vi "Facade 1.vi"(0 "Data In":T6, 2 "Display State In":T2={"Panels_Refnums_Array"=[], "Panel_Command"={"Operation"=enum."Add Item", "Data"=variant}}, 3 "Container State":T5) -> (6 "Data Out":T6, 7 "Display State Out":T2={"Panels_Refnums_Array"=[], "Panel_Command"={"Operation"=enum."Add Item", "Data"=variant}}, 8 "Action":T1)   [LabVIEW 2013, in "UI Panels.lvlib" / "Panels_XControl.xctl"]
uses:
  Panels_XControl.xctl
  Data 1.ctl
  <vilib>/_xctls/Container State.ctl
  State 1.ctl
  Controls/References/Panel_Refnums.ctl
  Controls/Panel_Command_Enum.ctl
  <vilib>/_xctls/Action.ctl
  Typedefs/Splitter Properties.ctl
  Typedefs/Menu Event.ctl
  <vilib>/_xctls/XControlSupport.lvlib
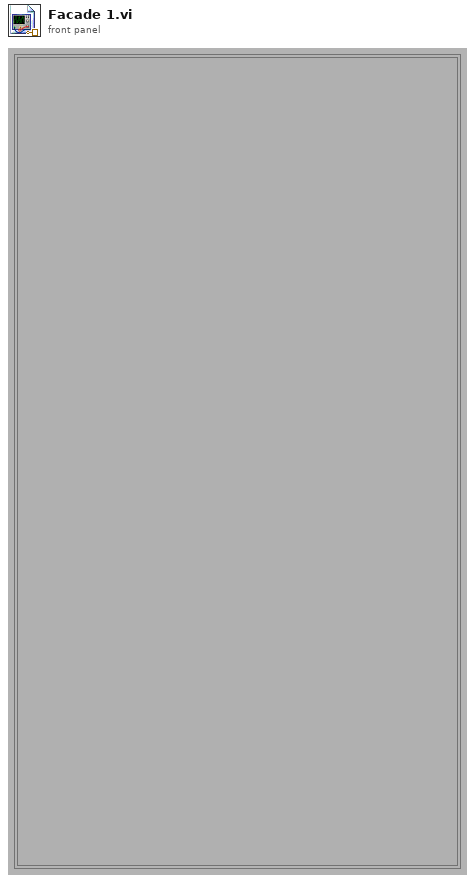
[diagram p1: front panel]
types:
  T1 = typedef "XControlSupport.lvlib/Action.ctl" = cluster{"Data Changed?":bool, "State Changed?":bool, "Action Name":string}
  T2 = typedef "UI Panels.lvlib/Panels_XControl.xctl/State 1.ctl" = cluster{"Panels_Refnums_Array":T3[], "Panel_Command":cluster{"Operation":T4, "Data":variant}}
  T3 = typedef "UI Panels.lvlib/Panels_XControl.xctl/Panel_Refnums.ctl" = cluster{"VI Refnum":refnum<vi>, "Command":refnum<user-event>, "Visible":bool}
  T4 = typedef "UI Panels.lvlib/Panels_XControl.xctl/Panel_Command_Enum.ctl" = enum16{"Idle", "Remove & Stop", "Add Item", "Delete Item", "Delete All", "Insert into Subpanel", "Register Menu Events", "Update Value", "Remove from Subpanel", "Set Title", "Set Menu Items", "Insert SubPanel", "Set Splitter Position", "Set Splitter Properties", "Add Menu Items"}
  T5 = typedef "XControlSupport.lvlib/Container State.ctl" = cluster{"Indicator?":bool, "Run Mode?":bool, " Refnum":refnum<vi>}
  T6 = typedef "UI Panels.lvlib/Panels_XControl.xctl/Data 1.ctl" = refnum<vi>[]
  T7 = typedef "UI Panels.lvlib/Panels_XControl.xctl/Splitter Properties.ctl" = cluster{"index":i32, "Height (Collapsed)":i32, "Height (Expanded)":i32, "Expanded by Default":bool, "Collapsable":bool, "Resizible":bool}
  T8 = typedef "UI Panels.lvlib/Panels_XControl.xctl/Menu Event.ctl" = refnum<user-event>
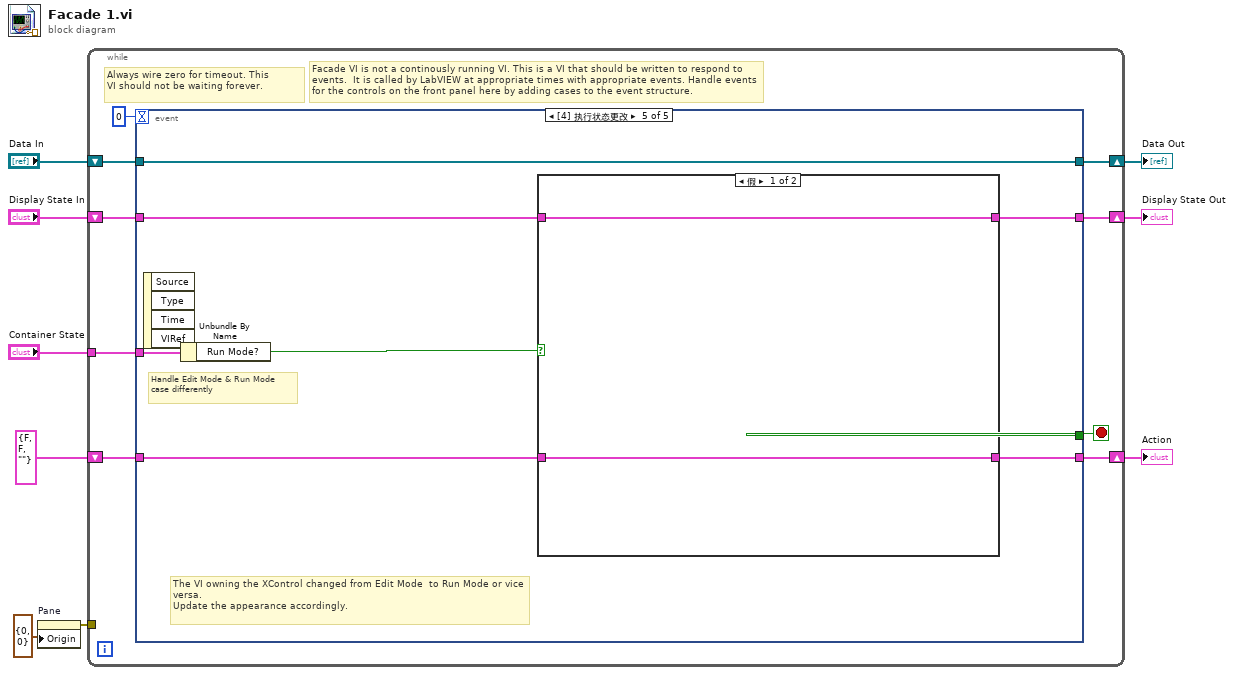
[diagram p0: block diagram]
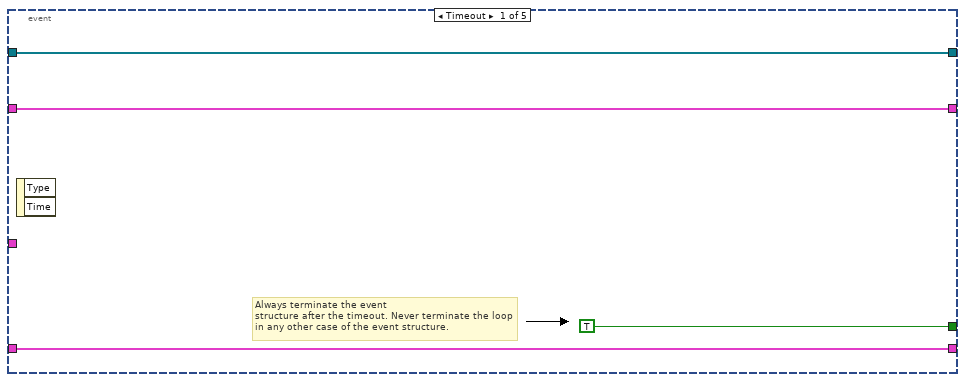
[diagram p2: hidden frame]
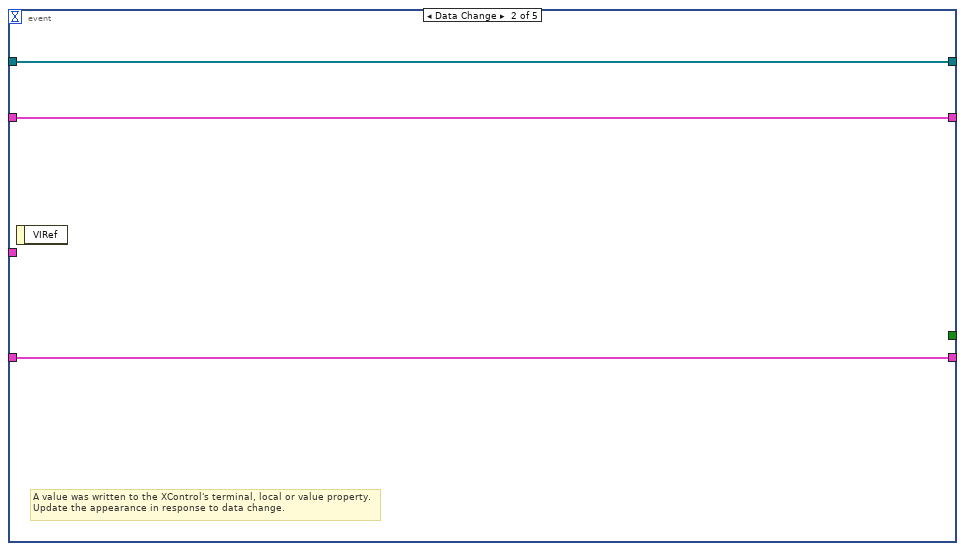
[diagram p3: hidden frame]
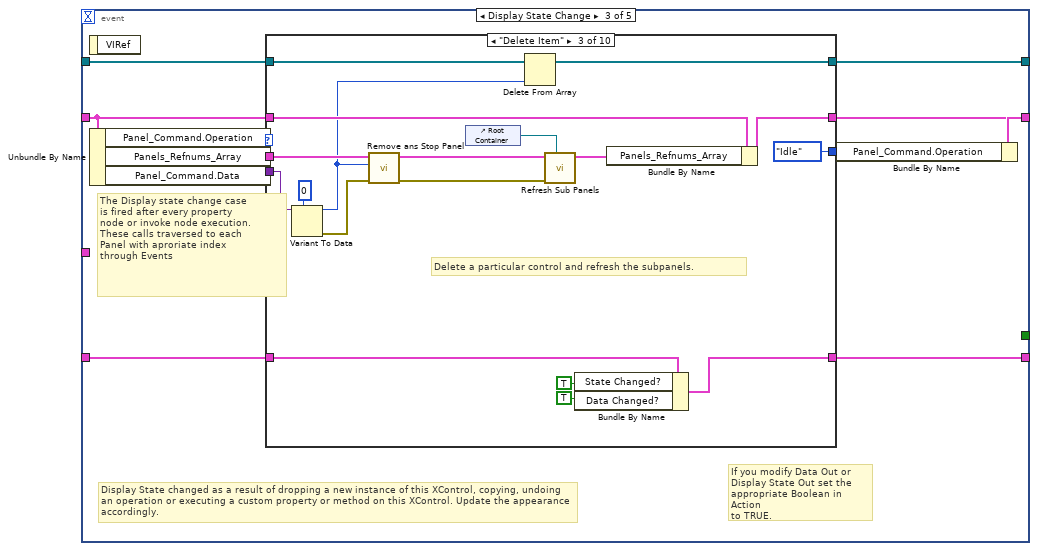
[diagram p4: hidden frame]
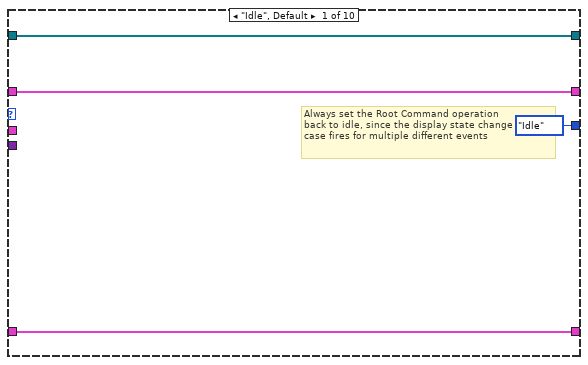
[diagram p5: hidden frame]
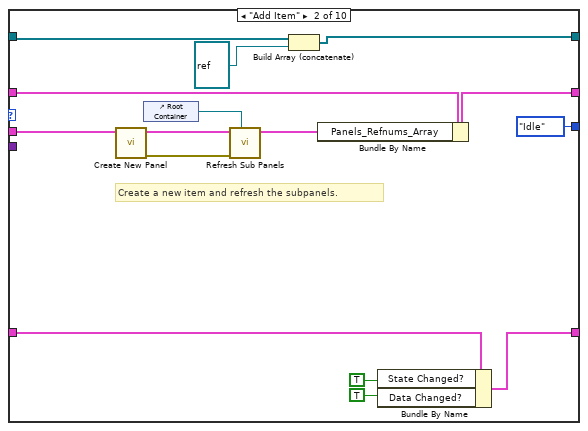
[diagram p6: hidden frame]
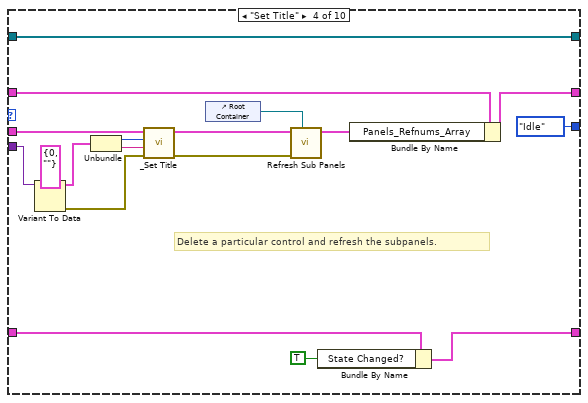
[diagram p7: hidden frame]
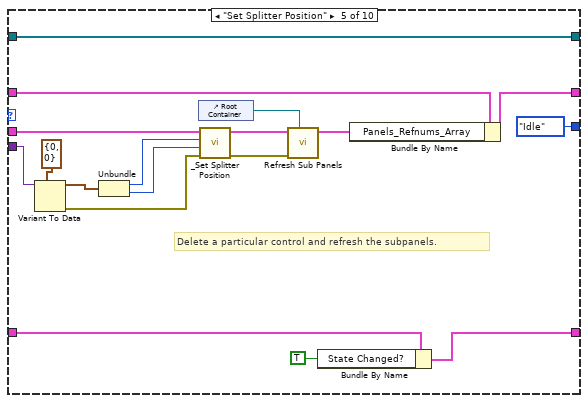
[diagram p8: hidden frame]
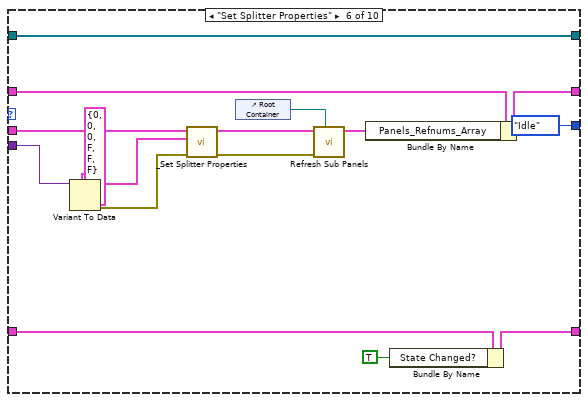
[diagram p9: hidden frame]
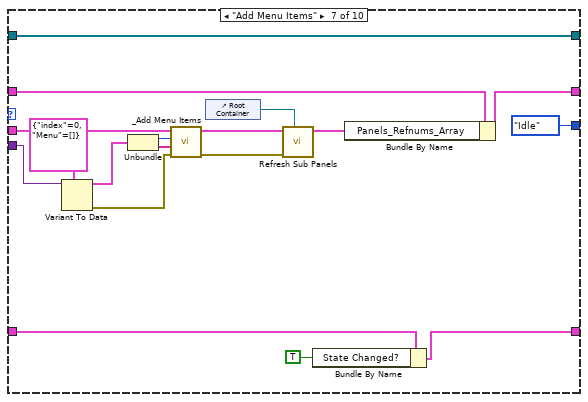
[diagram p10: hidden frame]
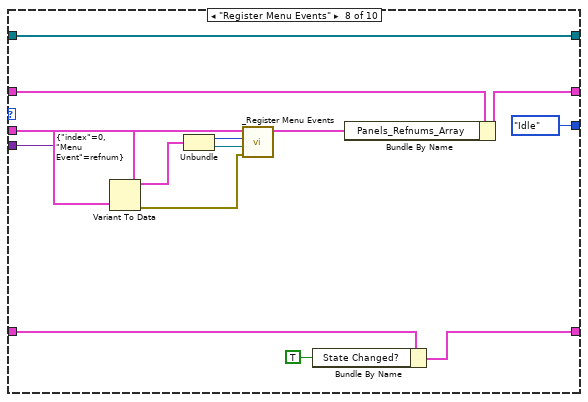
[diagram p11: hidden frame]
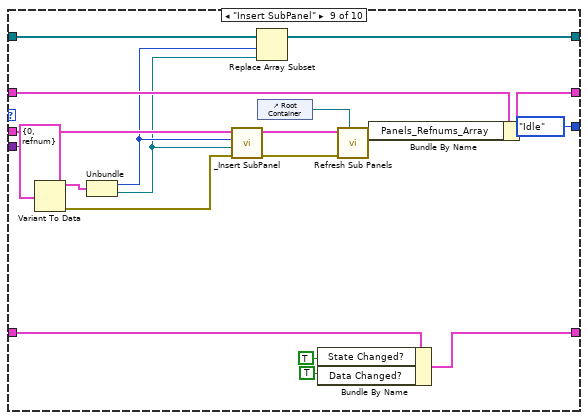
[diagram p12: hidden frame]
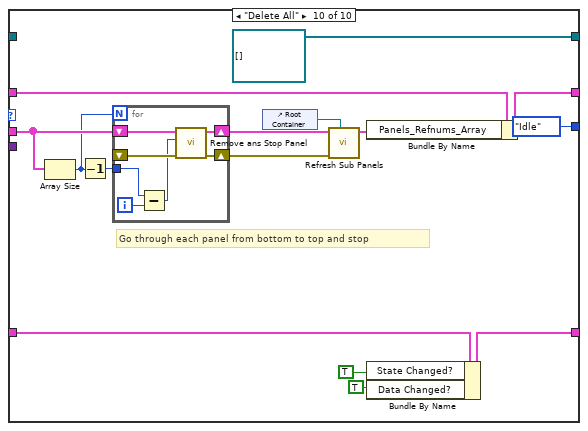
[diagram p13: hidden frame]
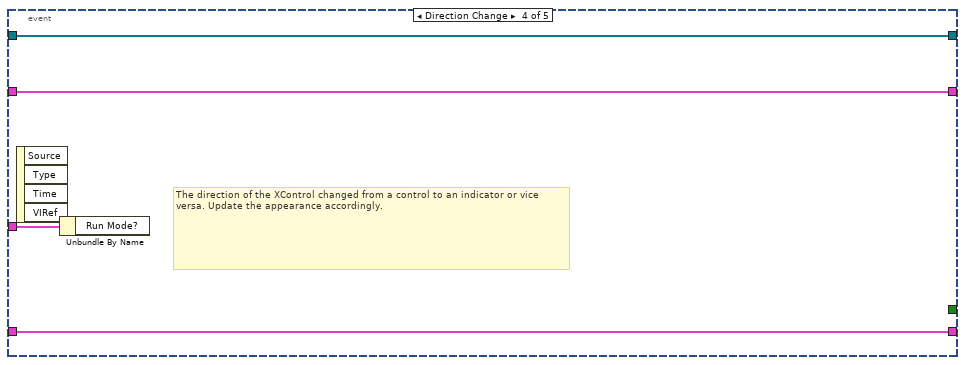
[diagram p14: hidden frame]
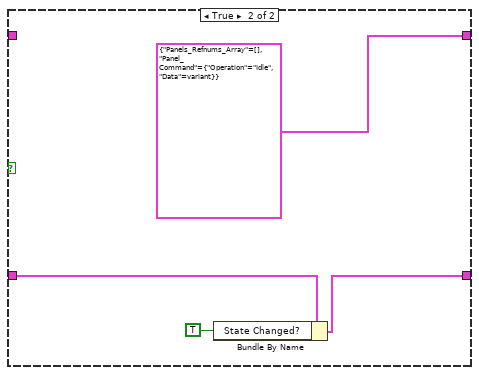
[diagram p15: hidden frame]
diagram:
  n1 = property on="Pane" class="Pane"("Origin"=cluster{"Horizontal":i16, "Vertical":i16} {"Horizontal"=0, "Vertical"=0}) -> (error out=w1:errorcluster)  [unwired: 2 in, 1 out]
  n2 = while {
    shift-right: [w17] -> w3
    shift-left: "Display State In" -> [w18]
    tunnel: "Container State" -> [w14]
    shift-right: [w12] -> w9
    shift-left: "Data In" -> [w13]
    shift-right: [w10] -> w5
    shift-left: T1 {"Data Changed?"=FALSE, "State Changed?"=FALSE, "Action Name"=""} ("Action") -> [w11]
    tunnel: w1 -> [_]
    stop <- w16 stop-if-true
    # "Facade VI is not a continously running VI. This is a VI that should be written to respond to events.  It is called by LabVIEW at appropriate times with appropriate events. Handle events for the controls on the front panel here by adding cases to the event structure."
    # "Always wire zero for timeout. This\nVI should not be waiting forever."
    n3 = event shown="[4] 执行状态更改" {
      selector: _ -> [_ _ _ _ _]
      dyn-events: _ -> [_ _ _ _ _]
      timeout: 0 -> [_ _ _ _ _]
      tunnel: w18 -> [w20 w24 w36 w203 w205]
      tunnel: [w20 w24 w32 w203 w207] -> w17
      tunnel: [TRUE _ _ _ _] -> w16
      tunnel: w14 -> [_ _ _ w204 w211]
      tunnel: w13 -> [w19 w25 w27 w202 w210]
      tunnel: [w19 w25 w26 w202 w210] -> w12
      tunnel: [w21 w23 w33 w201 w208] -> w10
      tunnel: w11 -> [w21 w23 w34 w201 w209]
      event Timeout {
        # "Always terminate the event\nstructure after the timeout. Never terminate the loop in any other case of the event structure."
        n4 = event-data() -> ()  [unwired: 3 out]
      }
      event Data Change {
        # "A value was written to the XControl's terminal, local or value property.\nUpdate the appearance in response to data change."
        n5 = event-data() -> ()  [unwired: 2 out]
      }
      event Display State Change {
        # "If you modify Data Out or\nDisplay State Out set the\nappropriate Boolean in Action\nto TRUE."
        # "The Display state change case\nis fired after every property\nnode or invoke node execution.\nThese calls traversed to each\nPanel with aproriate index\nthrough Events"
        # "Display State changed as a result of dropping a new instance of this XControl, copying, undoing an operation or executing a custom property or method on this XControl. Update the appearance accordingly."
        n6 = event-data() -> ()  [unwired: 2 out]
        n7 = Unbundle By Name(w36) -> ("Panel_Command.Operation"=w35:T4, "Panels_Refnums_Array"=w30:T3[], "Panel_Command.Data"=w29:variant)
        n8 = case shown="\"Delete Item\"" w35 {
          tunnel: w36 -> [w40 w55 w72 w91 w109 w120 w138 w156 w178 w188]
          tunnel: w34 -> [w39 w52 w70 w89 w107 w112 w134 w152 w176 w193]
          tunnel: [w40 w54 w71 w90 w108 w119 w137 w155 w177 w186] -> w31
          tunnel: [w39 w51 w68 w87 w105 w117 w135 w153 w174 w191] -> w33
          tunnel: w30 -> [_ w49 w65 w84 w102 w116 w133 w151 w171 w181]
          tunnel: w29 -> [_ _ w67 w86 w104 w115 w132 w150 w173 _]
          tunnel: [Panel_Command_Enum."Idle" ("Operation") Panel_Command_Enum."Idle" ("Operation") Panel_Command_Enum."Idle" ("Enum") Panel_Command_Enum."Idle" ("Enum") Panel_Command_Enum."Idle" ("Enum") Panel_Command_Enum."Idle" ("Operation") Panel_Command_Enum."Idle" ("Operation") Panel_Command_Enum."Idle" ("Operation") Panel_Command_Enum."Idle" ("Operation") Panel_Command_Enum."Idle" ("Operation")] -> w28
          tunnel: w27 -> [w37 w45 w60 w75 w93 w111 w127 w146 w164 _]
          tunnel: [w37 w43 w58 w75 w93 w111 w127 w146 w163 T6 [] ("Data In")] -> w26
          frame "Idle", Default {
            # "Always set the Root Command operation\nback to idle, since the display state change\ncase fires for multiple different events"
          }
          frame "Add Item" {
            # "Create a new item and refresh the subpanels."
            n9 = call "Create New Panel.vi"("Item_Refnums_Array In"=w49) -> ("error out"=w46:errorcluster, "Item_Refnums_Array Out"=w48:T3[])  [unwired: 1 in, 8 out]
            n10 = control-ref of="Root Container"() -> (w41:refnum<vi>)
            n11 = call "Refresh Sub Panels.vi"("Root Container"=w41, "error in (no error)"=w46, "Panels Refnums Array"=w48) -> ("Panels Refnums Array Out (dup)"=w47:T3[])  [unwired: 5 in, 3 out]
            n12 = Build Array (concatenate)(w45, refnum<vi> refnum ("VI Refnum")) -> (w43:T6)
            n13 = Bundle By Name(cluster=w55, "Panels_Refnums_Array"=w47) -> (w54:T2)
            n14 = Bundle By Name(cluster=w52, "State Changed?"=TRUE, "Data Changed?"=TRUE) -> (w51:T1)
          }
          frame "Delete Item" {
            # "Delete a particular control and refresh the subpanels."
            n15 = Variant To Data(type=0, Variant=w67) -> (data=w59:i32, error out=w64:errorcluster)  [unwired: 1 in]
            n16 = call "Remove ans Stop Panel.vi"("error in (no error)"=w64, "Index"=w59, "Item_Refnums_Array"=w65) -> ("error out"=w62:errorcluster, "Item_Refnums_Array Out"=w63:T3[])  [unwired: 2 in, 5 out]
            n17 = control-ref of="Root Container"() -> (w56:refnum<vi>)
            n18 = Delete From Array(array=w60, index=w59) -> (array with subset deleted=w58:T6)  [unwired: 1 in, 1 out]
            n19 = call "Refresh Sub Panels.vi"("Root Container"=w56, "error in (no error)"=w62, "Panels Refnums Array"=w63) -> ("Panels Refnums Array Out (dup)"=w61:T3[])  [unwired: 1 in, 7 out]
            n20 = Bundle By Name(cluster=w70, "State Changed?"=TRUE ("Data Changed?"), "Data Changed?"=TRUE) -> (w68:T1)
            n21 = Bundle By Name(cluster=w72, "Panels_Refnums_Array"=w61) -> (w71:T2)
          }
          frame "Set Title" {
            # "Delete a particular control and refresh the subpanels."
            n22 = Variant To Data(type=cluster{"index":i32, "New Title":string} {"index"=0, "New Title"=""} ("output cluster"), Variant=w86) -> (data=w78:cluster{"index":i32, "New Title":string}, error out=w83:errorcluster)  [unwired: 1 in]
            n23 = Unbundle(w78) -> ("index"=w77:i32, "New Title"=w76:string)
            n24 = call "_Set Title.vi"("error in (no error)"=w83, "Title"=w76, "Index"=w77, "Item_Refnums_Array"=w84) -> ("error out"=w81:errorcluster, "Item_Refnums_Array Out"=w82:T3[])  [unwired: 6 out]
            n25 = control-ref of="Root Container"() -> (w74:refnum<vi>)
            n26 = call "Refresh Sub Panels.vi"("Root Container"=w74, "error in (no error)"=w81, "Panels Refnums Array"=w82) -> ("Panels Refnums Array Out (dup)"=w80:T3[])  [unwired: 1 in, 7 out]
            n27 = Bundle By Name(cluster=w89, "State Changed?"=TRUE ("Data Changed?")) -> (w87:T1)
            n28 = Bundle By Name(cluster=w91, "Panels_Refnums_Array"=w80) -> (w90:T2)
          }
          frame "Set Splitter Position" {
            # "Delete a particular control and refresh the subpanels."
            n29 = Variant To Data(type=cluster{"index":i32, "index 2":i32} {"index"=0, "index 2"=0} ("output cluster"), Variant=w104) -> (data=w96:cluster{"index":i32, "index 2":i32}, error out=w101:errorcluster)  [unwired: 1 in]
            n30 = Unbundle(w96) -> ("index"=w95:i32, "index 2"=w94:i32)
            n31 = control-ref of="Root Container"() -> (w92:refnum<vi>)
            n32 = call "_Set Splitter Position.vi"("error in (no error)"=w101, "Position"=w94, "Index"=w95, "Item_Refnums_Array"=w102) -> ("error out"=w99:errorcluster, "Item_Refnums_Array Out"=w100:T3[])  [unwired: 6 out]
            n33 = call "Refresh Sub Panels.vi"("Root Container"=w92, "error in (no error)"=w99, "Panels Refnums Array"=w100) -> ("Panels Refnums Array Out (dup)"=w98:T3[])  [unwired: 1 in, 7 out]
            n34 = Bundle By Name(cluster=w107, "State Changed?"=TRUE ("Data Changed?")) -> (w105:T1)
            n35 = Bundle By Name(cluster=w109, "Panels_Refnums_Array"=w98) -> (w108:T2)
          }
          frame "Set Splitter Properties" {
            n36 = Variant To Data(type=T7 {"index"=0, "Height (Collapsed)"=0, "Height (Expanded)"=0, "Expanded by Default"=FALSE, "Collapsable"=FALSE, "Resizible"=FALSE} ("output cluster"), Variant=w115) -> (data=w113:T7, error out=w124:errorcluster)  [unwired: 1 in]
            n37 = call "_Set Splitter Properties.vi"("error in (no error)"=w124, "Splitter Properties"=w113, "Item_Refnums_Array"=w116) -> ("error out"=w122:errorcluster, "Item_Refnums_Array Out"=w123:T3[])  [unwired: 7 in]
            n38 = control-ref of="Root Container"() -> (w110:refnum<vi>)
            n39 = call "Refresh Sub Panels.vi"("Root Container"=w110, "error in (no error)"=w122, "Panels Refnums Array"=w123) -> ("Panels Refnums Array Out (dup)"=w121:T3[])  [unwired: 1 in, 7 out]
            n40 = Bundle By Name(cluster=w120, "Panels_Refnums_Array"=w121) -> (w119:T2)
            n41 = Bundle By Name(cluster=w112, "State Changed?"=TRUE ("Data Changed?")) -> (w117:T1)
          }
          frame "Add Menu Items" {
            n42 = Variant To Data(type=cluster{"index":i32, "Menu":string[]} {"index"=0, "Menu"=[]} ("output cluster"), Variant=w132) -> (data=w130:cluster{"index":i32, "Menu":string[]}, error out=w142:errorcluster)  [unwired: 1 in]
            n43 = Unbundle(w130) -> ("index"=w129:i32, "Menu"=w128:string[])
            n44 = call "_Add Menu Items.vi"("error in (no error)"=w142, "Menu Items"=w128, "Index"=w129, "Item_Refnums_Array"=w133) -> ("error out"=w140:errorcluster, "Item_Refnums_Array Out"=w141:T3[])  [unwired: 6 out]
            n45 = control-ref of="Root Container"() -> (w126:refnum<vi>)
            n46 = call "Refresh Sub Panels.vi"("Root Container"=w126, "error in (no error)"=w140, "Panels Refnums Array"=w141) -> ("Panels Refnums Array Out (dup)"=w139:T3[])  [unwired: 1 in, 7 out]
            n47 = Bundle By Name(cluster=w134, "State Changed?"=TRUE ("Data Changed?")) -> (w135:T1)
            n48 = Bundle By Name(cluster=w138, "Panels_Refnums_Array"=w139) -> (w137:T2)
          }
          frame "Register Menu Events" {
            n49 = Variant To Data(type=cluster{"index":i32, "Menu Event":T8} {"index"=0, "Menu Event"=refnum} ("output cluster"), Variant=w150) -> (data=w148:cluster{"index":i32, "Menu Event":T8}, error out=w157:errorcluster)  [unwired: 1 in]
            n50 = Unbundle(w148) -> ("index"=w147:i32, "Menu Event"=w144:T8)
            n51 = call "_Register Menu Events.vi"("error in (no error)"=w157, "Menu Event"=w144, "Index"=w147, "Item_Refnums_Array"=w151) -> ("Item_Refnums_Array Out"=w145:T3[])  [unwired: 6 in, 1 out]
            n52 = Bundle By Name(cluster=w152, "State Changed?"=TRUE ("Data Changed?")) -> (w153:T1)
            n53 = Bundle By Name(cluster=w156, "Panels_Refnums_Array"=w145) -> (w155:T2)
          }
          frame "Insert SubPanel" {
            n54 = Variant To Data(type=cluster{"index":i32, "VI Refnum":refnum<vi>} {"index"=0, "VI Refnum"=refnum} ("output cluster"), Variant=w173) -> (data=w165:cluster{"index":i32, "VI Refnum":refnum<vi>}, error out=w170:errorcluster)  [unwired: 1 in]
            n55 = Unbundle(w165) -> ("index"=w162:i32, "VI Refnum"=w161:refnum<vi>)
            n56 = call "_Insert SubPanel.vi"("error in (no error)"=w170, "VI Refnum"=w161, "Index"=w162, "Item_Refnums_Array"=w171) -> ("error out"=w168:errorcluster, "Item_Refnums_Array Out"=w169:T3[])  [unwired: 6 out]
            n57 = Replace Array Subset(array=w164, new element=w161, index=w162) -> (w163:T6)
            n58 = control-ref of="Root Container"() -> (w159:refnum<vi>)
            n59 = Bundle By Name(cluster=w176, "State Changed?"=TRUE ("Data Changed?"), "Data Changed?"=TRUE) -> (w174:T1)
            n60 = call "Refresh Sub Panels.vi"("Root Container"=w159, "error in (no error)"=w168, "Panels Refnums Array"=w169) -> ("Panels Refnums Array Out (dup)"=w167:T3[])  [unwired: 1 in, 7 out]
            n61 = Bundle By Name(cluster=w178, "Panels_Refnums_Array"=w167) -> (w177:T2)
          }
          frame "Delete All" {
            # "Go through each panel from bottom to top and stop"
            n62 = Array Size(array=w181) -> (size(s)=w179:i32)
            n63 = Decrement(x=w179) -> (x-1=w180:i32)
            n64 = for {
              N: w179 -> [_]
              shift-right: [w199] -> w190
              shift-left: w181 -> [w200]
              shift-right: [w198] -> w189
              shift-left: _ -> [w197]
              tunnel: w180 -> [w194]
              i -> [w196]
              n65 = Subtract(x=w194, y=w196) -> (x-y=w195:i32)
              n66 = call "Remove ans Stop Panel.vi"("error in (no error)"=w197, "Index"=w195, "Item_Refnums_Array"=w200) -> ("error out"=w198:errorcluster, "Item_Refnums_Array Out"=w199:T3[])  [unwired: 7 out]
            }
            n67 = control-ref of="Root Container"() -> (w182:refnum<vi>)
            n68 = call "Refresh Sub Panels.vi"("Root Container"=w182, "error in (no error)"=w189, "Panels Refnums Array"=w190) -> ("Panels Refnums Array Out (dup)"=w187:T3[])  [unwired: 1 in, 7 out]
            n69 = Bundle By Name(cluster=w188, "Panels_Refnums_Array"=w187) -> (w186:T2)
            n70 = Bundle By Name(cluster=w193, "State Changed?"=TRUE, "Data Changed?"=TRUE) -> (w191:T1)
          }
        }
        n71 = Bundle By Name(cluster=w31, "Panel_Command.Operation"=w28) -> (w32:T2)
      }
      event Direction Change {
        # "The direction of the XControl changed from a control to an indicator or vice versa. Update the appearance accordingly."
        n72 = event-data() -> ()  [unwired: 5 out]
        n73 = Unbundle By Name(w204) -> ()  [unwired: 1 out]
      }
      event Exec State Change {
        # "The VI owning the XControl changed from Edit Mode  to Run Mode or vice versa.\nUpdate the appearance accordingly."
        # "Handle Edit Mode & Run Mode\ncase differently"
        n74 = event-data() -> ()  [unwired: 5 out]
        n75 = Unbundle By Name(w211) -> ("Run Mode?"=w206:bool)
        n76 = case shown="假" w206 {
          tunnel: w209 -> [w212 w217]
          tunnel: [w212 w215] -> w208
          tunnel: [w213 T2 {"Panels_Refnums_Array"=[], "Panel_Command"={"Operation"=enum."Idle", "Data"=variant}} ("Display State In")] -> w207
          tunnel: w205 -> [w213 _]
          frame False {
          }
          frame True {
            n77 = Bundle By Name(cluster=w217, "State Changed?"=TRUE) -> (w215:T1)
          }
        }
      }
    }
  }
  "Display State Out" <- w3
  "Data Out" <- w9
  "Action" <- w5
